vi "SocketWhile.vi"(8 "error out":errorcluster, 10 "socket 2":T1={"端口"=10013, "timeout"=10013, "标准差倍数"=0.0, "address"="{\"ad\":1}", "abnormal"="{\"ad\":0}"}, 11 "SocketQueue":T2) -> (4 "socket":string="连接成功")   [LabVIEW 2018]
uses:
  Initialize/CreateQueue/SocketQueue.ctl
  socket.ctl
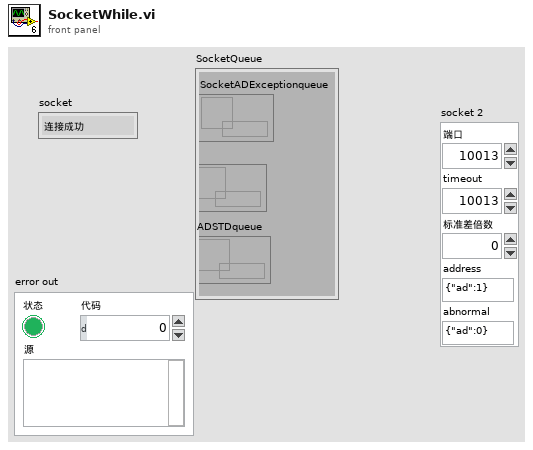
[diagram p1: front panel]
types:
  T1 = typedef "socket.ctl" = cluster{"端口":u16, "timeout":u16, "标准差倍数":dbl, "address":string, "abnormal":string}
  T2 = typedef "SocketQueue.ctl" = cluster{"ADSTDqueue ":refnum<queue>, "SocketADExceptionqueue":refnum<queue>, "  SocketAD":refnum<queue>}
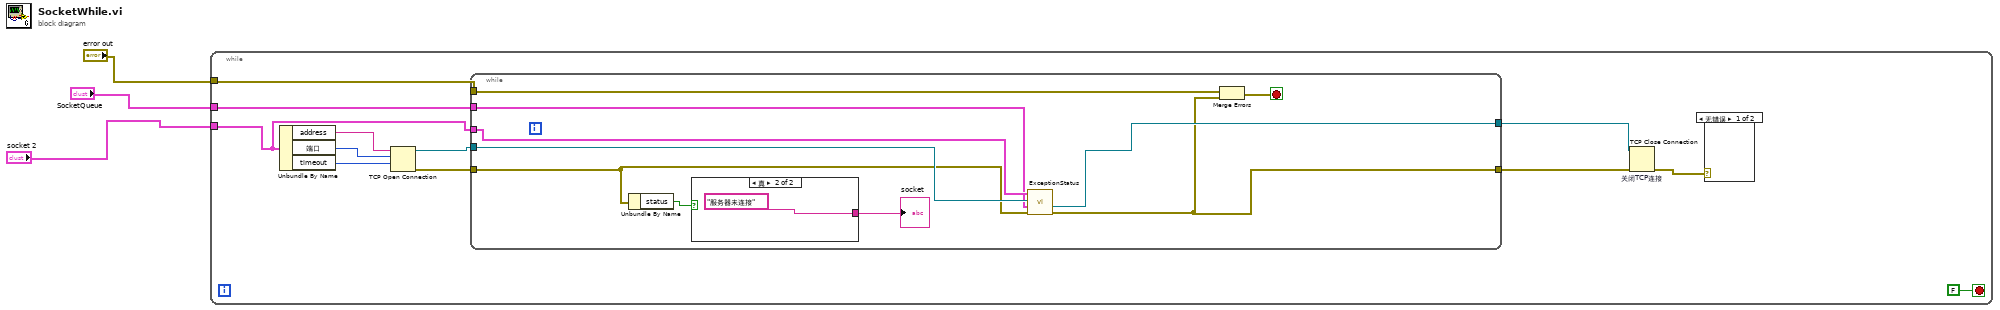
[diagram p0: block diagram]
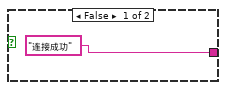
[diagram p3: hidden frame]
diagram:
  n1 = while {
    tunnel: "error out" -> [w15]
    tunnel: "socket 2" -> [w6]
    tunnel: "SocketQueue" -> [w4]
    stop <- FALSE stop-if-true
    n2 = Unbundle By Name(w6) -> ("address"=w5:string, "端口"=w10:u16, "timeout"=w9:u16)
    n3 = TCP Open Connection(address=w5, remote port or service name=w10, timeout ms (60000)=w9) -> (connection ID=w13:refnum<k5>, error out=w14:errorcluster)  [unwired: 2 in]
    n4 = while {
      tunnel: w13 -> [w20]
      tunnel: [w18] -> w11
      tunnel: w14 -> [w19]
      tunnel: [w17] -> w12
      tunnel: w15 -> [w23]
      tunnel: w6 -> [w21]
      tunnel: w4 -> [w16]
      stop <- w24 stop-if-true
      n5 = Unbundle By Name(w19) -> ("status"=w25:bool)
      n6 = case shown="真" w25 {
        tunnel: ["连接成功" "服务器未连接" ("文本.文本")] -> w22
        frame False {
        }
        frame True {
        }
      }
      "socket" <- w22
      n7 = call "ExceptionStatus.vi"("错误输入（无错误）"=w19, "SocketQueue"=w16, "connection ID输入"=w20, "socket 2"=w21) -> ("错误输出"=w17:errorcluster, "connection ID输出"=w18:refnum<k5>)  [unwired: 6 in]
      n8 = Merge Errors(w23, w17) -> (w24:errorcluster)
    }
    n9 = TCP Close Connection "关闭TCP连接"(connection ID=w11, error in (no error)=w12) -> (error out=w8:errorcluster)  [unwired: 2 out]
    n10 = case shown="无错误" w8 {
      frame No Error {
      }
      frame Error {
      }
    }
  }
